vi "RollUntil.vi"() -> ()   [LabVIEW 2014]
panel:
  out "Roll Value History":i32(graph)
  in  "Die N Sides":i32=6
  out "Roll Number":i32
  out "Complete Roll History":i32[](array[numeric])
  in  "Target Roll":i32=4
  # "Roll a virtual die until it equals a specified value"
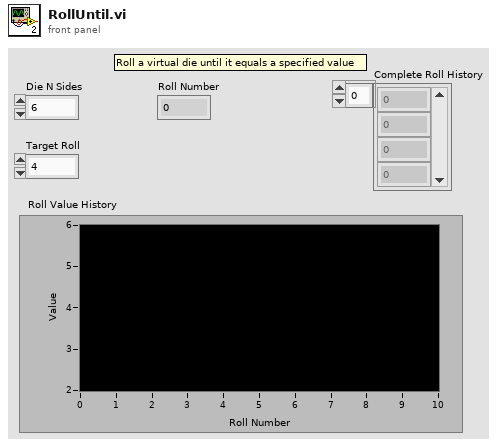
[diagram p1: front panel]
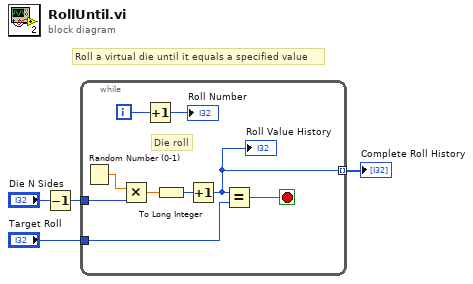
[diagram p0: block diagram]
diagram:
  # "Roll a virtual die until it equals a specified value"
  n1 = Decrement(x="Die N Sides") -> (x-1=w1:i32)
  n2 = while {
    tunnel: "Target Roll" -> [w11]
    tunnel: [w6] -> w3 mode=indexing
    tunnel: w1 -> [w7]
    i -> [w9]
    stop <- w12 stop-if-true
    # "Die roll"
    n3 = Random Number (0-1)() -> (number: 0 to 1=w13:dbl)
    n4 = Multiply(x=w13, y=w7) -> (x*y=w5:dbl)
    n5 = Increment(x=w9) -> (x+1=→"Roll Number":i32)
    n6 = To Long Integer(number=w5) -> (32bit integer=w10:i32)
    n7 = Increment(x=w10) -> (x+1=w6:i32)
    "Roll Value History" <- w6
    n8 = Equal?(x=w6, y=w11) -> (x = y?=w12:bool)
  }
  "Complete Roll History" <- w3
